vi "swish.vi"(2 "Z":dbl) -> (0 "Swish(Z)":dbl)   [LabVIEW 2020]
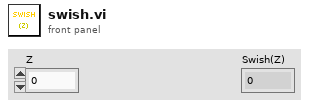
[diagram p1: front panel]
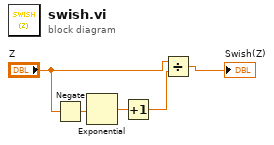
[diagram p0: block diagram]
diagram:
  n1 = Negate(x="Z") -> (-x=w2:dbl)
  n2 = Exponential(1:w2) -> (0:w3:dbl)
  n3 = Increment(x=w3) -> (x+1=w4:dbl)
  n4 = Divide(x="Z", y=w4) -> (x/y=→"Swish(Z)":dbl)
